vi "Counter_Reset.vi"(0 "Error In":errorcluster, 3 "Control":string) -> (1 "CounterDevRef out":T1, 2 "Error Out":errorcluster)   [LabVIEW 2016]
uses:
  <vilib>/Rock Robotics/WPI/Counter/WPI_CounterDevRef.ctl
  <vilib>/Rock Robotics/SystemInterfaces/Counter/FPGA_CounterCtrSystemIndex.ctl
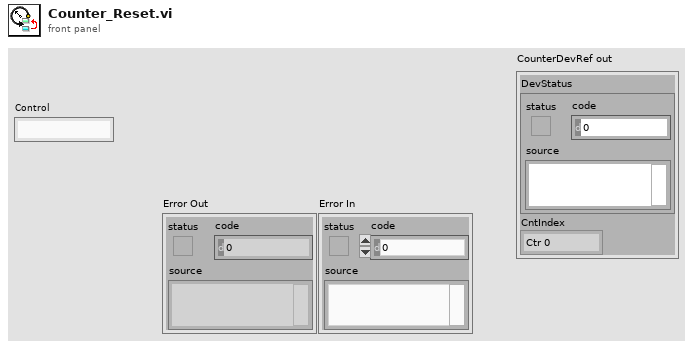
[diagram p1: front panel]
types:
  T1 = typedef "WPI_CounterDevRef.ctl" = cluster{"DevStatus":errorcluster, "CntIndex":T2}
  T2 = typedef "FPGA_CounterCtrSystemIndex.ctl" = enum8{"Ctr 0", "Ctr 1", "Ctr 2", "Ctr 3", "Ctr 4", "Ctr 5", "Ctr 6", "Ctr 7", "Invalid"}
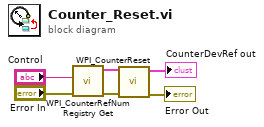
[diagram p0: block diagram]
diagram:
  n1 = call <vilib>:"WPI_CounterRefNum Registry Get.vi"("error in (no error)"="Error In", "refnum name"="Control") -> ("error out"=w6:errorcluster, "CounterDevRef"=w5:T1)  [unwired: 8 in]
  n2 = call <vilib>:"WPI_CounterReset.vi"("error in (no error)"=w6, "CounterDevRef in"=w5) -> ("error out"=→"Error Out":errorcluster, "CounterDevRef out"=→"CounterDevRef out":T1)  [unwired: 8 in]
